vi "Pockels-Make sequence array length even.vi"(11 "Single line AO sequence in":dbl[](array[numeric])) -> (3 "Single line AO sequence out":dbl[](array[numeric]))   [LabVIEW 2020]
uses:
  <vilib>/GPower/Comparison/Library/IsOdd/IsOddI32.vi
  <vilib>/GPower/Comparison/GPComparison.lvlib
panel:
  out "Output length":i32
  out "Input length":i32
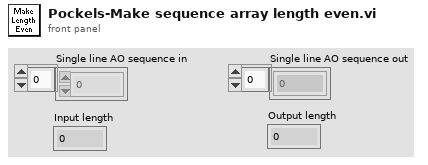
[diagram p1: front panel]
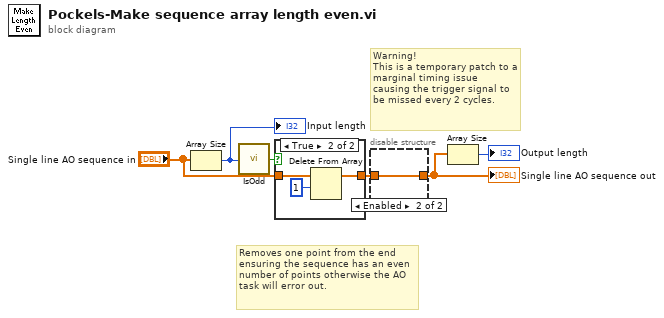
[diagram p0: block diagram]
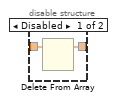
[diagram p2: hidden frame]
diagram:
  # "Warning!\nThis is a temporary patch to a marginal timing issue \ncausing the trigger signal to be missed every 2 cycles."
  # "Removes one point from the end ensuring the sequence has an even number of points otherwise the AO task will error out."
  n1 = Array Size(array="Single line AO sequence in") -> (size(s)=w1:i32)
  "Input length" <- w1
  n2 = call-poly <vilib>:"IsOdd.vi"("x"=w1) -> ("Odd?"=w4:bool)  [unwired: 4 in]
  n3 = case shown="True" w4 {
    tunnel: "Single line AO sequence in" -> [w7 w10]
    tunnel: [w7 w9] -> w5
    frame False {
    }
    frame True {
      n4 = Delete From Array(array=w10, length=1) -> (array with subset deleted=w9:dbl[])  [unwired: 1 in, 1 out]
    }
  }
  n5 = disable-structure "Diagram Disable Structure" shown="Enabled" {
    disable-tunnel: w5 -> [w12 w13]
    disable-tunnel: [w11 w13] -> w2
    frame Disabled {
      n6 = Delete From Array(array=w12) -> (array with subset deleted=w11:dbl[])  [unwired: 2 in, 1 out]
    }
    frame Enabled {
    }
  }
  "Single line AO sequence out" <- w2
  n7 = Array Size(array=w2) -> (size(s)=→"Output length":i32)
